vi "AbsolutePosition_KCubeDCServo.vi"(6 "set absolute position":dbl, 7 "lower limit":dbl, 9 "upper limit":dbl, 10 "go to button":bool, 11 ".NET Refnum in":refnum<k24>) -> (0 "get absolute position":dbl, 3 "absolute position response limit":string)   [LabVIEW 2019]
doc: "Set, get, and run absolute positions. Along with stage limit responses can be set."
uses:
  D:/Victor Sun/optical trap control/Kinesis/ThorLabs.MotionControl.KCube.DCServoCLI.dll
  Kinesis/ThorLabs.MotionControl.KCube.DCServoCLI.dll
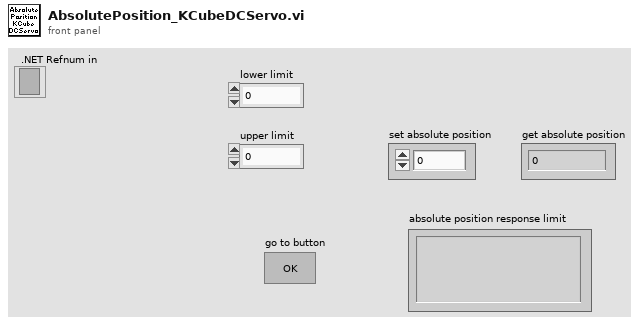
[diagram p1: front panel]
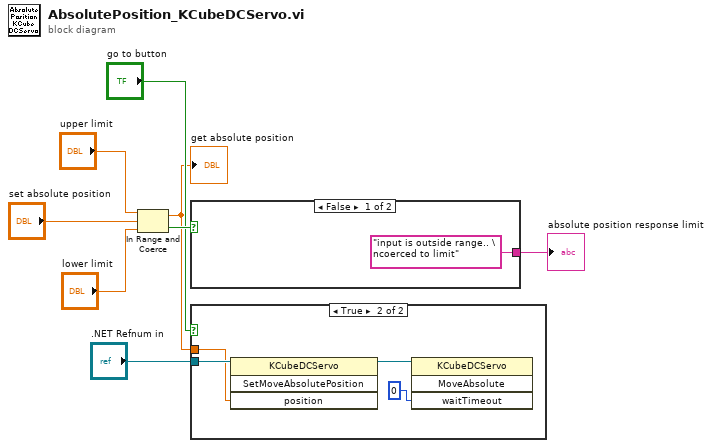
[diagram p0: block diagram]
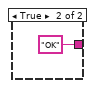
[diagram p2: hidden frame]
diagram:
  n1 = In Range and Coerce(upper limit="upper limit", x="set absolute position", lower limit="lower limit") -> (coerced(x)=w1:dbl, In Range?=w8:bool)
  "get absolute position" <- w1
  n2 = case shown="False" w8 {
    tunnel: ["input is outside range.. \ncoerced to limit" ("INPUT RESPONSE ERROR") "OK" ("INPUT RESPONSE ERROR")] -> w7
    frame False {
    }
    frame True {
    }
  }
  "absolute position response limit" <- w7
  n3 = case shown="True" "go to button" {
    tunnel: ".NET Refnum in" -> [_ w14]
    tunnel: w1 -> [_ w13]
    frame False {
    }
    frame True {
      n4 = invoke class="KCubeDCServo" method="SetMoveAbsolutePosition"(reference=w14, "position"=w13) -> (reference out=w12:refnum<k24>)  [unwired: 2 in, 3 out]
      n5 = invoke class="KCubeDCServo" method="MoveAbsolute"(reference=w12, "waitTimeout"=0) -> ()  [unwired: 2 in, 4 out]
    }
  }
